vi "Initialize Sessions - NSess.vi"(6 "initialize and close session behavior":T2, 7 "visa open timeout":u32, 8 "error in":errorcluster, 9 "access mode":T1 items=["VISA Defaults"=0, "Exclusive Lock"=1, "Load Configured Settings"=4], 10 "instrument type id":string, 11 "session reservation in":refnum<class "Session Reservation.lvclass">) -> (0 "error out":errorcluster, 1 "channel lists":string[](array[string]), 2 "sessions":refnum<visa-resource-name>[](array[refnum]), 3 "session reservation out":refnum<class "Session Reservation.lvclass">)   [LabVIEW 2020, in "VISA Sessions.lvlib"]
doc: "Create the VISA sessions from the <b>session reservation in</b> and the <b>instrument type id</b>. The <b>instrument type id</b> must match the Instrument Type Id for the custom VISA instrument in the pin map."
uses:
  VISA Sessions.lvlib
  b3cb301c-7684-4518-818f-a956a366db36.vi
  Session Factory/Session Factory.lvclass
  APIs/Session Management V1/Session Reservation/Session Reservation.lvclass
  APIs/Session Management V1/Session Reservation/Initialize and Close Session Behavior.ctl
  <vilib>/Instr/_visa.llb/VISA Open Access Mode.ctl
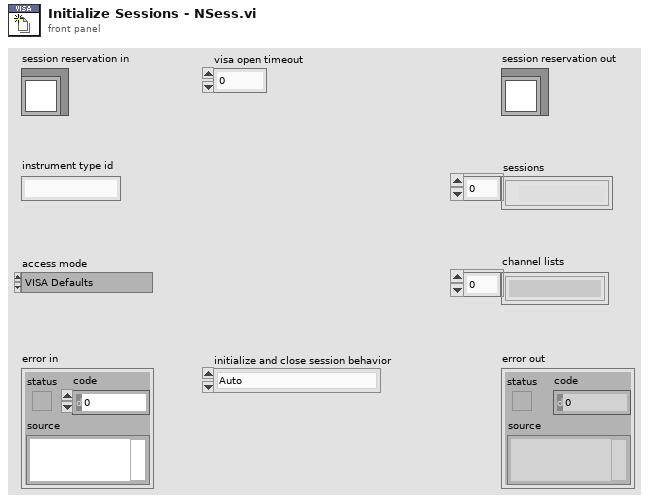
[diagram p1: front panel]
types:
  T1 = typedef "VISA Open Access Mode.ctl" = u32
  T2 = typedef "Plug-In SDK Session Management V1.lvlib/Session Reservation.lvclass/Initialize and Close Session Behavior.ctl" = enum16{"Auto", "Initialize and Close", "Attach and Detach", "Initialize and Detach", "Attach and Close"}
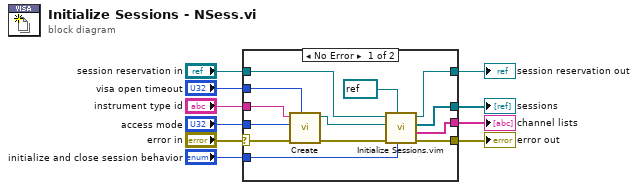
[diagram p0: block diagram]
diagram:
  n1 = case shown="No Error" "error in" {
    selector: "error in" -> [w22 w25]
    tunnel: [w18 w25] -> w9
    tunnel: [w20 w24] -> w7
    tunnel: "session reservation in" -> [w21 w24]
    tunnel: "instrument type id" -> [w23 _]
    tunnel: [w17 _] -> w5
    tunnel: [w16 _] -> w4
    tunnel: "initialize and close session behavior" -> [w14 _]
    tunnel: "visa open timeout" -> [w12 _]
    tunnel: "access mode" -> [w11 _]
    frame No Error {
      n2 = call "Create.vi"("visa open timeout"=w12, "error in"=w22, "access mode"=w11, "instrument type id"=w23) -> ("error out"=w19:errorcluster, "session factory out"=w15:refnum<class "Session Factory.lvclass">)  [unwired: 6 in]
      n3 = call "Initialize Sessions.vim"("initialize and close session behavior"=w14, "session type"=refnum<visa-resource-name> refnum ("VISA resource name out"), "error in"=w19, "session factory"=w15, "session reservation in"=w21) -> ("error out"=w18:errorcluster, "channel lists"=w16:string[], "sessions"=w17:refnum<visa-resource-name>[], "session reservation out"=w20:refnum<class "Session Reservation.lvclass">)  [unwired: 3 in]
    }
    frame Error {
    }
  }
  "error out" <- w9
  "session reservation out" <- w7
  "sessions" <- w5
  "channel lists" <- w4
